vi "_Palette_.vi"   [LabVIEW 2020]
uses:
  UI_Actor/UI_Actor/UI_Actor.lvclass
  UI_Actor/UI_Actor Messages/UI_Resize Msg/UI_Resize Msg.lvclass
  UI_Actor/UI_Actor Messages/UI_Hide Msg/UI_Hide Msg.lvclass
  UI_Actor/UI_Actor Messages/UI_ShowIn_FreeWindow Msg/UI_ShowIn_FreeWindow Msg.lvclass
  UI_Actor/UI_Actor Messages/UI_ShowIn_Subpanel Msg/UI_ShowIn_Subpanel Msg.lvclass
  UI_Actor/UI_Actor Messages/Ping Tree Msg/Ping Tree Msg.lvclass
  UI_Actor/UI_Actor Messages/UI_KBB_Trig Msg/UI_KBB_Trig Msg.lvclass
  UI_Actor/UI_Actor/ctl_UE_Msg.ctl
  support/Databox.lvlibp/TypesTools/Data/Data.lvclass
  support/Databox.lvlibp/TypesTools/Config/Config.lvclass
  UI_Actor/UI_Actor/ctl_InternalMapItem.ctl
  UI_Actor/UI_Actor Messages/UI_AutoRefresh Msg/UI_AutoRefresh Msg.lvclass
  support/Databox.lvlibp/Databox_sealed/Databox_sealed.lvclass
  UI_Actor/UI_Actor/UI_Elmts_Reads[Labels]-DBL.vi
types:
  T1 = typedef "UI_Actor.lvlib/UI_Actor.lvclass/ctl_InternalMapItem.ctl" = cluster{"Config":refnum<class "Config.lvclass">, "LatestData":refnum<class "Data.lvclass">}
  T2 = typedef "UI_Actor.lvlib/UI_Actor.lvclass/ctl_UE_Msg.ctl" = cluster{"Cmd":string, "Payload":string}
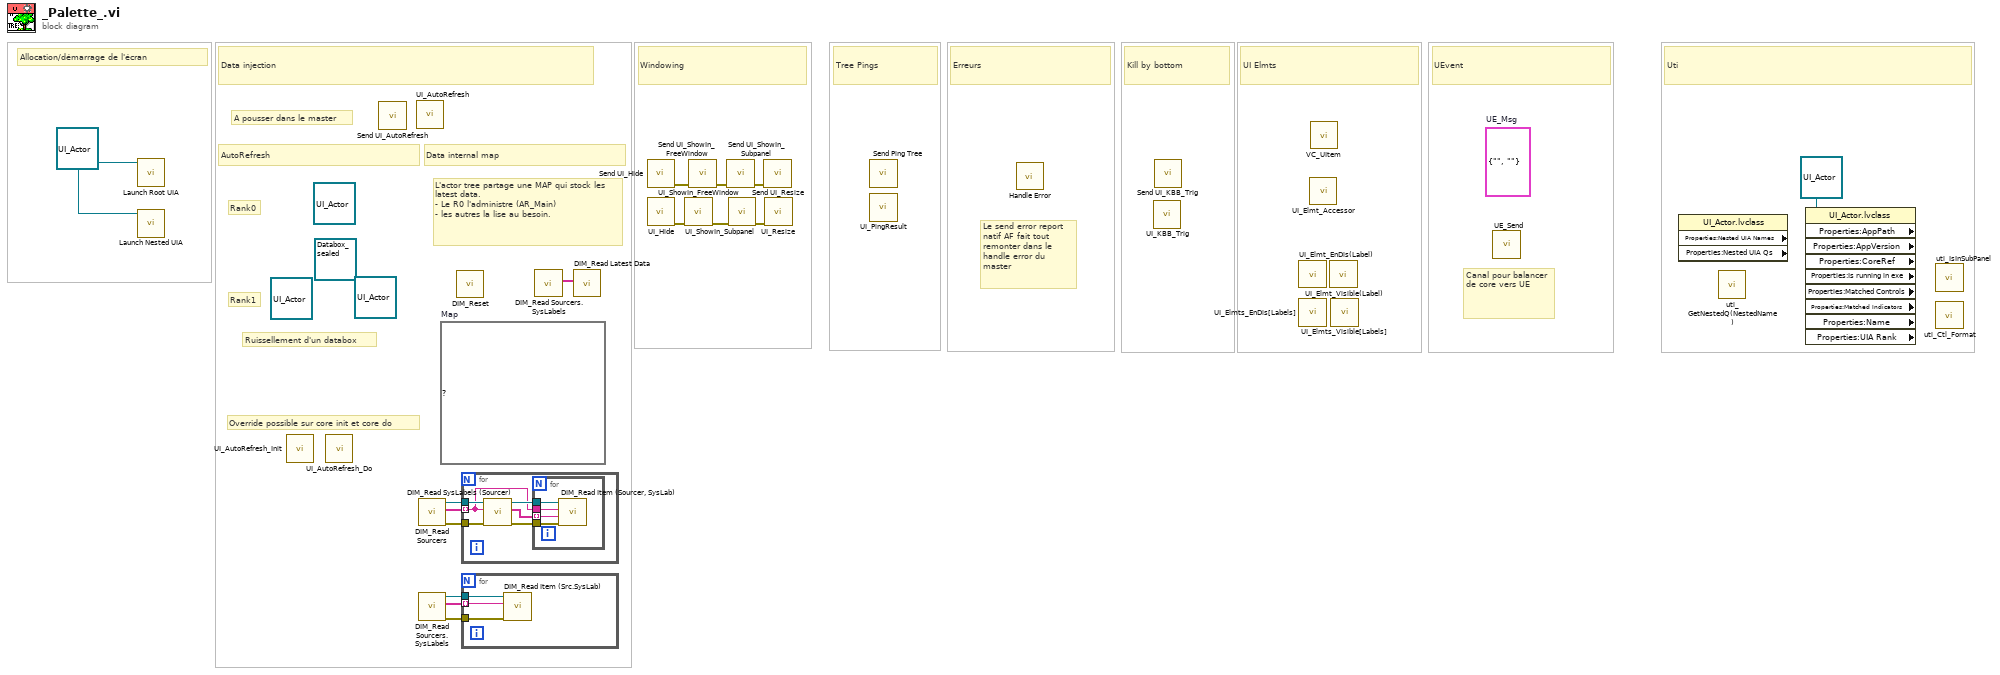
[diagram p0: block diagram]
diagram:
  (unwired) map{string, map{string, T1}} {}  # Map
  (unwired) refnum<class "Databox_sealed.lvclass"> refnum ("Databox.lvlibp:Databox_sealed.lvclass")
  (unwired) refnum<class "UI_Actor.lvclass"> refnum ("UI_Actor.lvlib:UI_Actor.lvclass")
  (unwired) refnum<class "UI_Actor.lvclass"> refnum ("UI_Actor.lvlib:UI_Actor.lvclass")
  (unwired) refnum<class "UI_Actor.lvclass"> refnum ("UI_Actor.lvlib:UI_Actor.lvclass")
  (unwired) T2 {"Cmd"="", "Payload"=""}  # UE_Msg
  w15 = refnum<class "UI_Actor.lvclass"> refnum ("UI_Actor.lvlib:UI_Actor.lvclass")
  # "Le send error report natif AF fait tout remonter dans le handle error du master"
  # "Override possible sur core init et core do"
  # "Data internal map"
  # "Ruissellement d'un databox"
  # "A pousser dans le master"
  # "AutoRefresh"
  # "L'actor tree partage une MAP qui stock les latest data.\n- Le R0 l'administre (AR_Main)\n- les autres la lise au besoin."
  # "Rank1"
  # "Rank0"
  # "Canal pour balancer de core vers UE"
  # "UEvent"
  # "Uti"
  # "UI Elmts"
  # "Kill by bottom"
  # "Erreurs"
  # "Tree Pings"
  # "Windowing"
  # "Data injection"
  # "Allocation/démarrage de l'écran"
  n1 = call "Launch Root UIA.vi"("UI_Actor in"=w15) -> ()  [unwired: 9 in, 2 out]
  n2 = call "Launch Nested UIA.vi"("Caller UIA in"=w15) -> ()  [unwired: 8 in, 3 out]
  n3 = call-dynamic "UI_AutoRefresh_Init.vi"() -> ()  [unwired: 10 in, 2 out]
  n4 = call-dynamic "UI_AutoRefresh_Do.vi"() -> ()  [unwired: 10 in, 2 out]
  n5 = call "Send UI_AutoRefresh.vi"() -> ()  [unwired: 10 in, 2 out]
  n6 = call "UI_AutoRefresh.vi"() -> ()  [unwired: 10 in, 2 out]
  n7 = call "DIM_Read Sourcers.vi"() -> ("error out"=w4:errorcluster, "DIM Sourcers"=w6:string[], "UI_Actor out"=w5:refnum<class "UI_Actor.lvclass">)  [unwired: 9 in]
  n8 = call "DIM_Read Sourcers.SysLabels.vi"() -> ("error out"=w1:errorcluster, "DIM Sourcer.SysLabels"=w3:string[], "UI_Actor out"=w2:refnum<class "UI_Actor.lvclass">)  [unwired: 9 in]
  n9 = call "DIM_Reset.vi"() -> ()  [unwired: 10 in, 2 out]
  n10 = for {
    tunnel: w6 -> [w17] mode=indexing
    tunnel: w5 -> [w21]
    tunnel: w4 -> [w20]
    n11 = call "DIM_Read SysLabels (Sourcer).vi"("error in (no error)"=w20, "Sourcer"=w17, "UI_Actor in"=w21) -> ("error out"=w18:errorcluster, "DIM Sourcer's SysLabels"=w16:string[], "UI_Actor out"=w19:refnum<class "UI_Actor.lvclass">)  [unwired: 6 in]
    n12 = for {
      tunnel: w19 -> [w25]
      tunnel: w18 -> [w24]
      tunnel: w17 -> [w23]
      tunnel: w16 -> [w22] mode=indexing
      n13 = call "DIM_Read Item (Sourcer, SysLab).vi"("error in (no error)"=w24, "SysLabel"=w22, "Sourcer"=w23, "UI_Actor in"=w25) -> ()  [unwired: 4 in, 4 out]
    }
  }
  n14 = for {
    tunnel: w3 -> [w28] mode=indexing
    tunnel: w2 -> [w27]
    tunnel: w1 -> [w26]
    n15 = call "DIM_Read Item (Src.SysLab).vi"("error in (no error)"=w26, "Sourcer.SysLabel"=w28, "UI_Actor in"=w27) -> ()  [unwired: 5 in, 4 out]
  }
  n16 = call "DIM_Read Sourcers.SysLabels.vi"() -> ("DIM Sourcer.SysLabels"=w7:string[])  [unwired: 9 in, 2 out]
  n17 = call "DIM_Read Latest Data.vi"("Src.SysLabels"=w7) -> ()  [unwired: 8 in, 3 out]
  n18 = call "Send UI_Hide.vi"() -> ("error out"=w10:errorcluster)  [unwired: 10 in, 1 out]
  n19 = call-dynamic "UI_Hide.vi"() -> ("error out"=w13:errorcluster)  [unwired: 10 in, 1 out]
  n20 = call-dynamic "UI_ShowIn_FreeWindow.vi"("error in (no error)"=w13) -> ("error out"=w12:errorcluster)  [unwired: 9 in, 1 out]
  n21 = call "Send UI_ShowIn_FreeWindow.vi"("error in (no error)"=w10) -> ("error out"=w9:errorcluster)  [unwired: 9 in, 1 out]
  n22 = call "Send UI_ShowIn_Subpanel.vi"("error in (no error)"=w9) -> ("error out"=w8:errorcluster)  [unwired: 9 in, 1 out]
  n23 = call-dynamic "UI_ShowIn_Subpanel.vi"("error in (no error)"=w12) -> ("error out"=w11:errorcluster)  [unwired: 9 in, 1 out]
  n24 = call "Send UI_Resize.vi"("error in (no error)"=w8) -> ()  [unwired: 9 in, 2 out]
  n25 = call-dynamic "UI_Resize.vi"("error in (no error)"=w11) -> ()  [unwired: 9 in, 2 out]
  n26 = call "Send Ping Tree.vi"() -> ()  [unwired: 10 in, 2 out]
  n27 = call-dynamic "UI_PingResult.vi"() -> ()  [unwired: 10 in, 2 out]
  n28 = call-dynamic "Handle Error.vi"() -> ()  [unwired: 9 in, 3 out]
  n29 = call-dynamic "UI_KBB_Trig.vi"() -> ()  [unwired: 10 in, 2 out]
  n30 = call "Send UI_KBB_Trig.vi"() -> ()  [unwired: 10 in, 2 out]
  n31 = call "UI_Elmt_EnDis(Label).vi"() -> ()  [unwired: 9 in, 3 out]
  n32 = call "UI_Elmts_EnDis[Labels].vi"() -> ()  [unwired: 9 in, 3 out]
  n33 = call-poly "UI_Elmt_Accessor.vi"() -> ()  [unwired: 8 in, 4 out]
  n34 = call-dynamic "VC_UItem.vi"() -> ()  [unwired: 10 in, 2 out]
  n35 = call "UI_Elmt_Visible(Label).vi"() -> ()  [unwired: 9 in, 3 out]
  n36 = call "UI_Elmts_Visible[Labels].vi"() -> ()  [unwired: 9 in, 3 out]
  n37 = call "UE_Send.vi"() -> ()  [unwired: 10 in, 2 out]
  n38 = property class="UI_Actor.lvclass" props=["Properties:Nested UIA Names", "Properties:Nested UIA Qs"]() -> ()  [unwired: 2 in, 4 out]
  n39 = call "uti_GetNestedQ(NestedName).vi"() -> ()  [unwired: 9 in, 3 out]
  n40 = property class="UI_Actor.lvclass" props=["Properties:AppPath", "Properties:AppVersion", "Properties:CoreRef", "Properties:Is running in exe", "Properties:Matched Controls", "Properties:Matched Indicators", "Properties:Name", "Properties:UIA Rank"](reference=refnum<class "UI_Actor.lvclass"> refnum ("UI_Actor in")) -> ()  [unwired: 1 in, 10 out]
  n41 = call "uti_IsInSubPanel.vi"() -> ()  [unwired: 9 in, 3 out]
  n42 = call "uti_Ctl_Format.vi"() -> ()  [unwired: 10 in, 2 out]
